vi "humidity sensor.vi"() -> ()   [LabVIEW 2022 SP3]
uses:
  <vilib>/MakerHub/LINX/LMH-LINX.lvlib
  <vilib>/MakerHub/LINX/Public/Utilities/Open Serial.vi
panel:
  in  "Serial Port":refnum<visa-resource-name>="N/A"
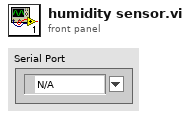
[diagram p1: front panel]
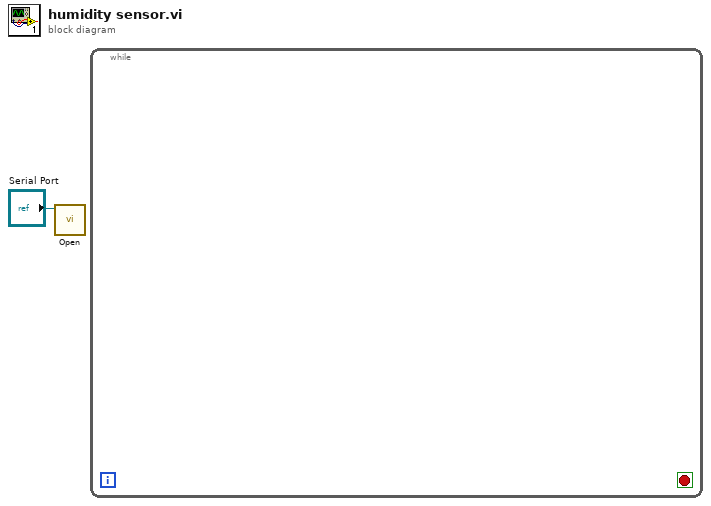
[diagram p0: block diagram]
diagram:
  n1 = call-poly <vilib>:"Open.vi"("Serial Port"="Serial Port") -> ()  [unwired: 8 in, 3 out]
  n2 = while {
    stop <- _ stop-if-true
  }
